vi "Drawing Pad.vi"(8 "错误输入":errorcluster) -> (0 "错误输出":errorcluster, 3 "图像数据":cluster{"红色":u8, "绿色":u8, "蓝色":u8}[][](array[cluster]))   [LabVIEW 2012]
uses:
  <vilib>/Utility/cursorutil.llb/Set Cursor (Icon Pict).vi
panel:
  in  "清除":bool
  in  "画笔颜色":u32(colorbox)
  in  "完成":bool
  out "图片":picture
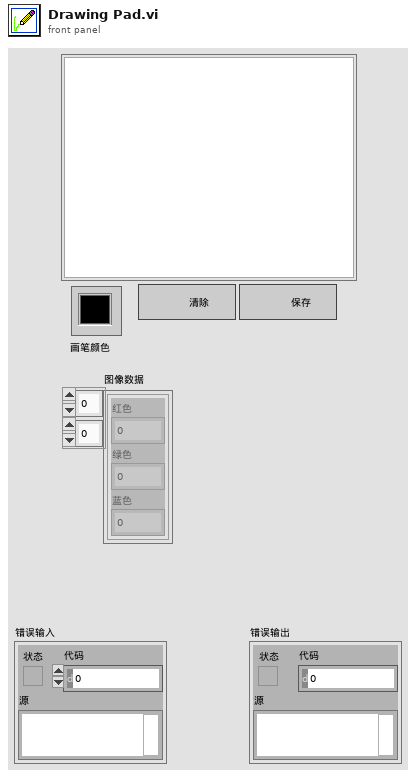
[diagram p1: front panel]
types:
  T1 = typedef "LVPoint32TypeDef.ctl" = cluster{"Horizontal":i32, "Vertical":i32}
  T2 = typedef "LVBoundsTypeDef.ctl" = cluster{"Width":u32, "Height":u32}
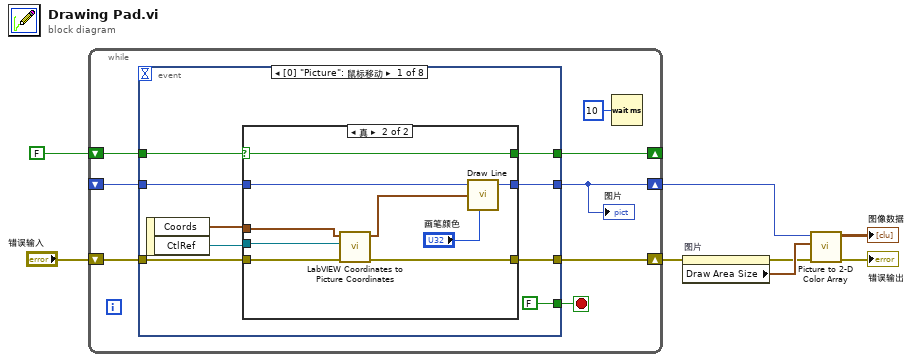
[diagram p0: block diagram]
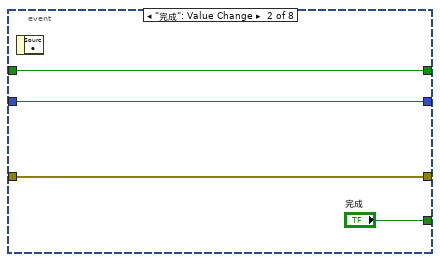
[diagram p3: hidden frame]
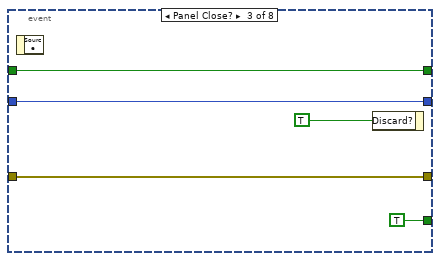
[diagram p4: hidden frame]
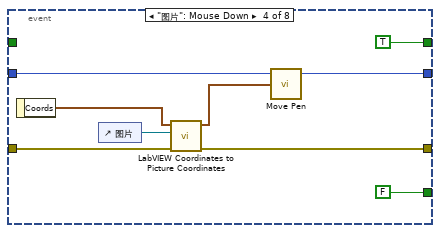
[diagram p5: hidden frame]
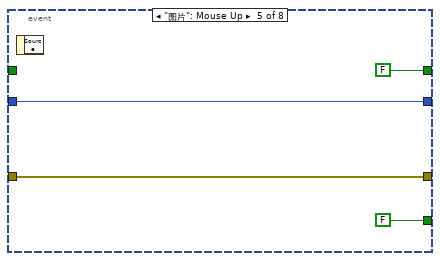
[diagram p6: hidden frame]
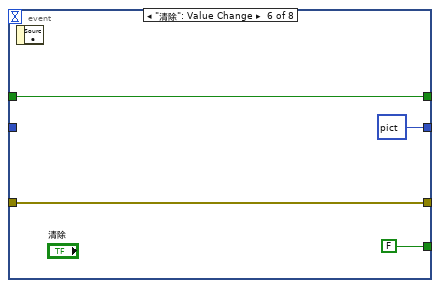
[diagram p7: hidden frame]
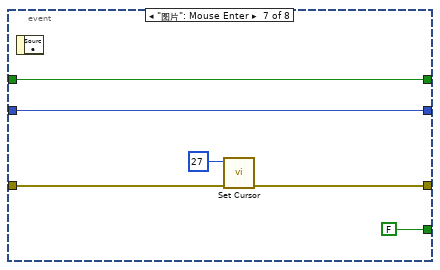
[diagram p8: hidden frame]
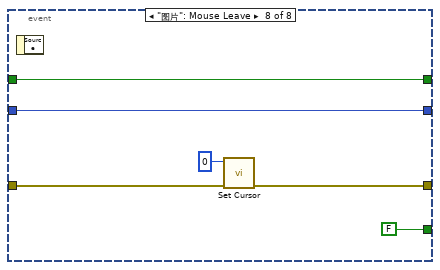
[diagram p9: hidden frame]
diagram:
  n1 = while {
    shift-right: [w14] -> _
    shift-left: FALSE -> [w16]
    shift-right: [w13] -> w2
    shift-left: "错误输入" -> [w12]
    shift-right: [w10] -> w5
    shift-left: _ -> [w11]
    stop <- w15 stop-if-true
    n2 = event shown="[0] \"Picture\": 鼠标移动" {
      selector: _ -> [_ _ _ _ _ _ _ _]
      dyn-events: _ -> [_ _ _ _ _ _ _ _]
      timeout: _ -> [_ _ _ _ _ _ _ _]
      tunnel: w16 -> [w25 w40 w46 _ _ w62 w65 w72]
      tunnel: [FALSE ("完成") "完成" TRUE ("完成") FALSE FALSE FALSE ("完成") FALSE ("完成") FALSE ("完成")] -> w15
      tunnel: [w24 w40 w46 TRUE FALSE w62 w65 w72] -> w14
      tunnel: [w18 w38 w44 w48 w56 w61 w68 w74] -> w13
      tunnel: w12 -> [w19 w38 w44 w49 w56 w61 w67 w73]
      tunnel: [w23 w39 w45 w50 w57 picture data[5B] ("新图片") w66 w71] -> w10
      tunnel: w11 -> [w22 w39 w45 w51 w57 _ w66 w71]
      event "图片": Mouse Move {
        n3 = event-data ("事件数据节点")() -> ("Coords"=w21:T1, "CtlRef"=w20:refnum<vi>)  [unwired: 1 in]
        n4 = case shown="真" w25 {
          selector: w25 -> [w28 w37]
          tunnel: [w28 w37] -> w24
          tunnel: [w27 w36] -> w23
          tunnel: w22 -> [w27 w35]
          tunnel: w21 -> [_ w30]
          tunnel: w20 -> [_ w31]
          tunnel: w19 -> [w26 w33]
          tunnel: [w26 w32] -> w18
          frame False {
          }
          frame True {
            n5 = call "LabVIEW Coordinates to Picture Coordinates.vi"("错误输入"=w33, "控件引用"=w31, "LabVIEW坐标"=w30) -> ("错误输出"=w32:errorcluster, "图片控件坐标"=w29:cluster{"水平":i32, "垂直":i32})  [unwired: 7 in]
            n6 = call <vilib>:"Draw Line.vi"("picture"=w35, "end point"=w29, "color(black)"="画笔颜色") -> ("new picture"=w36:picture)  [unwired: 6 in]
          }
        }
      }
      event "完成": Value Change {
        n7 = event-data ("事件数据节点")() -> ()  [unwired: 1 in, 1 out]
      }
      event Panel Close? {
        n8 = event-data ("事件数据节点")() -> ()  [unwired: 1 in, 1 out]
        n9 = event-data ("事件过滤节点")("Discard?"=TRUE ("放弃？")) -> ()  [unwired: 1 in, 1 out]
      }
      event "图片": Mouse Down {
        n10 = event-data ("事件数据节点")() -> ("Coords"=w53:T1)  [unwired: 1 in]
        n11 = control-ref of="图片"() -> (w52:refnum<vi>)
        n12 = call "LabVIEW Coordinates to Picture Coordinates.vi"("错误输入"=w49, "控件引用"=w52, "LabVIEW坐标"=w53) -> ("错误输出"=w48:errorcluster, "图片控件坐标"=w47:cluster{"水平":i32, "垂直":i32})  [unwired: 7 in]
        n13 = call <vilib>:"Move Pen.vi"("new position"=w47, "picture"=w51) -> ("new picture"=w50:picture)  [unwired: 3 in]
      }
      event "图片": Mouse Up {
        n14 = event-data ("事件数据节点")() -> ()  [unwired: 1 in, 1 out]
      }
      event "清除": Value Change {
        n15 = event-data ("事件数据节点")() -> ()  [unwired: 1 in, 1 out]
      }
      event "图片": Mouse Enter {
        n16 = event-data ("事件数据节点")() -> ()  [unwired: 1 in, 1 out]
        n17 = call-poly <vilib>:"Set Cursor.vi"("error in (no error)"=w67, "icon"=u16 27 ("图标")) -> ("error out"=w68:errorcluster)  [unwired: 8 in, 1 out]
      }
      event "图片": Mouse Leave {
        n18 = event-data ("事件数据节点")() -> ()  [unwired: 1 in, 1 out]
        n19 = call-poly <vilib>:"Set Cursor.vi"("error in (no error)"=w73, "icon"=u16 0 ("图标")) -> ("error out"=w74:errorcluster)  [unwired: 8 in, 1 out]
      }
    }
    "图片" <- w10
    n20 = Wait (ms) ("等待(ms)")(milliseconds to wait=u32 10 ("等待时间（毫秒）")) -> ()  [unwired: 1 out]
  }
  n21 = property on="图片" class="Pict"(error in=w2) -> (error out=w1:errorcluster, "Draw Area Size"=w3:T2)  [unwired: 1 in, 1 out]
  n22 = call "Picture to 2-D Color Array.vi"("错误输入"=w1, "输入簇"=w3, "图片"=w5) -> ("错误输出"=→"错误输出":errorcluster, "颜色数组"=→"图像数据":cluster{"红色":u8, "绿色":u8, "蓝色":u8}[][])  [unwired: 7 in]
